vi "InsertHorizontalLine.vi"(8 "error in (no error)":errorcluster, 10 "ParentTag":string, 11 "Menu in":refnum<class "MGI_ToolStrip.lvclass">) -> (0 "error out":errorcluster, 3 "Menu out":refnum<class "MGI_ToolStrip.lvclass">)   [LabVIEW 2019, in "MGI_ToolStrip.lvclass"]
doc: "Inserts a horizontal line into the menu. Called when a MenuSeparatorItem is added.\n\nAuthored by Derek E. Trepanier\nsupport@mooregoodideas.com\nwww.mooregoodideas.com\n\nCopyright (c) 2012, Moore Good Ideas, Inc.\n\nAll rights reserved.\n\nRedistribution and use in source and binary forms, with or without modification, are permitted provided that the following conditions are met:\n\n * Redistributions of source code must retain the above copyright notice, this list of conditions and the following disclaimer.\n * Redistributions in binary form must reproduce the above copyright notice, this list of conditions and the following disclaimer in the documentation and/or other materials provided with the distribution.\n * Neither the name of Moore Good Ideas, Inc. nor the names of its contributors may be used to endorse or promote products derived from this software without specific prior written permission.\n\nTHIS SOFTWARE IS PROVIDED BY THE COPYRIGHT HOLDERS AND CONTRIBUTORS \"AS IS\" AND ANY EXPRESS OR IMPLIED WARRANTIES, INCLUDING, BUT NOT LIMITED TO, THE IMPLIED WARRANTIES OF MERCHANTABILITY AND FITNESS FOR A PARTICULAR PURPOSE ARE DISCLAIMED. IN NO EVENT SHALL THE COPYRIGHT OWNER OR CONTRIBUTORS BE LIABLE FOR ANY DIRECT, INDIRECT, INCIDENTAL, SPECIAL, EXEMPLARY, OR CONSEQUENTIAL DAMAGES (INCLUDING, BUT NOT LIMITED TO, PROCUREMENT OF SUBSTITUTE GOODS OR SERVICES; LOSS OF USE, DATA, OR PROFITS; OR BUSINESS INTERRUPTION) HOWEVER CAUSED AND ON ANY THEORY OF LIABILITY, WHETHER IN CONTRACT, STRICT LIABILITY, OR TORT (INCLUDING NEGLIGENCE OR OTHERWISE) ARISING IN ANY WAY OUT OF THE USE OF THIS SOFTWARE, EVEN IF ADVISED OF THE POSSIBILITY OF SUCH DAMAGE."
uses:
  MGI_ToolStrip.lvclass
  MGI_ToolStrip.lvclass/MGI_ToolStrip.ctl
  System.Windows.Forms
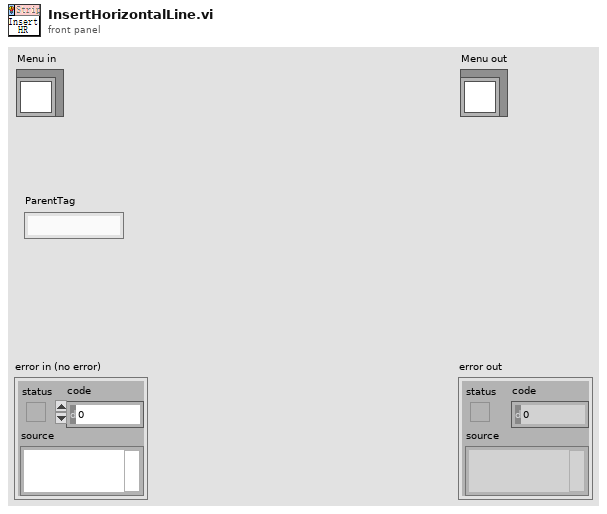
[diagram p1: front panel]
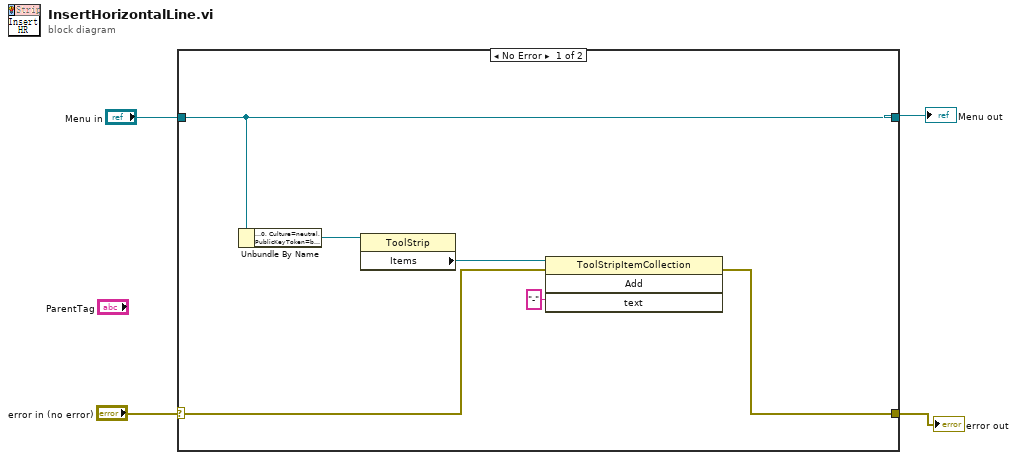
[diagram p0: block diagram]
diagram:
  n1 = case shown="No Error" "error in (no error)" {
    selector: "error in (no error)" -> [w6 w11]
    tunnel: "Menu in" -> [w9 w12]
    tunnel: [w9 w12] -> w3
    tunnel: [w5 w11] -> w1
    frame No Error {
      n2 = Unbundle By Name(w9) -> ("ToolStrip"=w8:refnum<k24>)
      n3 = property class="ToolStrip"(reference=w8) -> ("Items"=w7:refnum<k24>)  [unwired: 1 in, 2 out]
      n4 = invoke class="ToolStripItemCollection" method="Add"(reference=w7, error in=w6, "text"="-") -> (error out=w5:errorcluster)  [unwired: 1 in, 3 out]
    }
    frame Error {
    }
  }
  "error out" <- w1
  "Menu out" <- w3
